vi "PS Control (FPGA).vi"() -> ()   [LabVIEW 2019]
uses:
  <vilib>/eio/EIONode/EIONode.xnode
  <vilib>/rvi/eio/common/nirviEmuTemplateMethod_errors.vi
panel:
  out "Actual Loop Time":u32
  in  "Loop Timer (uSec)":u32=10000
  in  "PS Enable 4":bool
  in  "PS Enable 3":bool
  in  "PS Enable 2":bool
  in  "PS Enable 1":bool
  out "PS Feedback 4":fxp<+/-,24,5>
  out "PS Feedback 3":fxp<+/-,24,5>
  out "PS Feedback 2":fxp<+/-,24,5>
  out "PS Feedback 1":fxp<+/-,24,5>
  in  "PS CMD 4":fxp<+/-,20,5>
  in  "PS CMD 3":fxp<+/-,20,5>
  in  "PS CMD 2":fxp<+/-,20,5>
  in  "PS CMD 1":fxp<+/-,20,5>
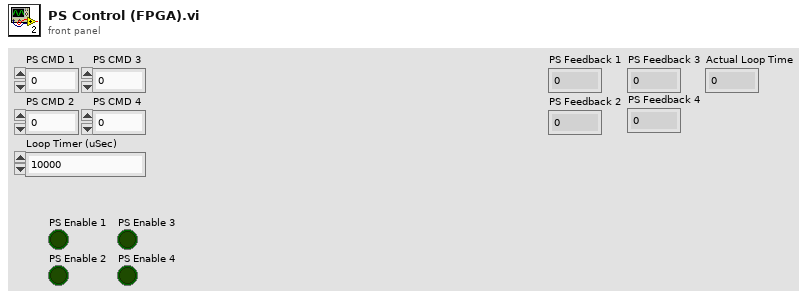
[diagram p1: front panel]
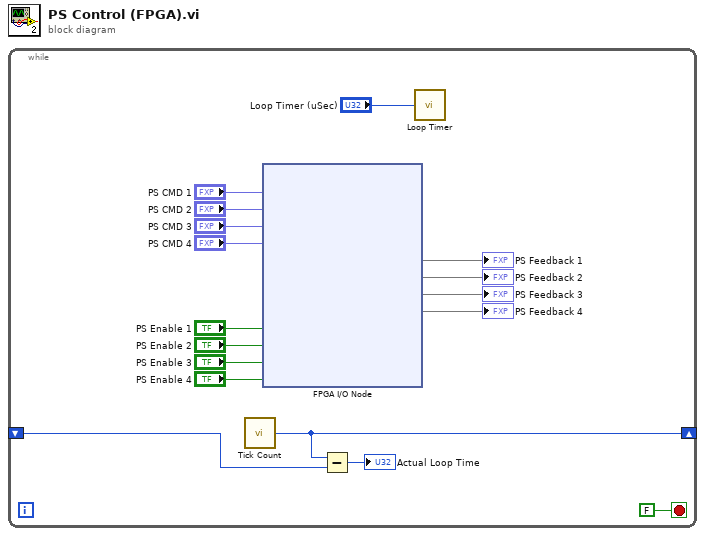
[diagram p0: block diagram]
diagram:
  n1 = while {
    shift-right: [w3] -> _
    shift-left: _ -> [w2]
    stop <- FALSE stop-if-true
    n2 = call "Tick Count"() -> ("Tick Count(uSec)"=w3:u32)
    n3 = xnode "FPGA I/O Node"("AO0"="PS CMD 1", "AO1"="PS CMD 2", "AO2"="PS CMD 3", "AO3"="PS CMD 4", "RMC/DIO0"="PS Enable 1", "RMC/DIO1"="PS Enable 2", "RMC/DIO2"="PS Enable 3", "RMC/DIO3"="PS Enable 4") -> ("Speed_Current_1 (AI0)"=→"PS Feedback 1", "Speed_Current_2 (AI1)"=→"PS Feedback 2", "Speed_Current_3 (AI2)"=→"PS Feedback 3", "Speed_Current_4 (AI3)"=→"PS Feedback 4")  [unwired: 12 in, 12 out]
    n4 = Subtract(x=w3, y=w2) -> (x-y=→"Actual Loop Time":u32)
    n5 = call "Loop Timer"("Count(uSec)"="Loop Timer (uSec)") -> ()  [unwired: 1 out]
  }
